vi "Manhattan Distance.vi"(10 "To":T1, 11 "From":T1) -> (3 "Manhattan Distance":i32)   [LabVIEW 2020, in "SquareBattle.lvlib"]
uses:
  SquareBattle.lvlib
  Position.ctl
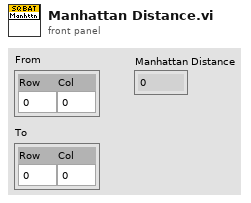
[diagram p1: front panel]
types:
  T1 = typedef "SquareBattle.lvlib/Position.ctl" = cluster{"Row":i32, "Col":i32}
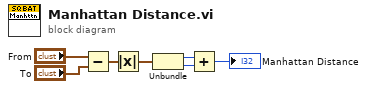
[diagram p0: block diagram]
diagram:
  n1 = Subtract(x="From", y="To") -> (x-y=w5:T1)
  n2 = Absolute Value(x=w5) -> (abs(x)=w4:T1)
  n3 = Unbundle(w4) -> ("Row"=w3:i32, "Col"=w2:i32)
  n4 = Add(x=w3, y=w2) -> (x+y=→"Manhattan Distance":i32)
